vi "Setting_Command_List.vi"(8 "error in (no error)":errorcluster, 11 "VISA resource name":refnum<visa-resource-name>) -> (0 "error out":errorcluster, 2 "read buffer":string, 3 "VISA resource name out":refnum<visa-resource-name>)   [LabVIEW 2020]
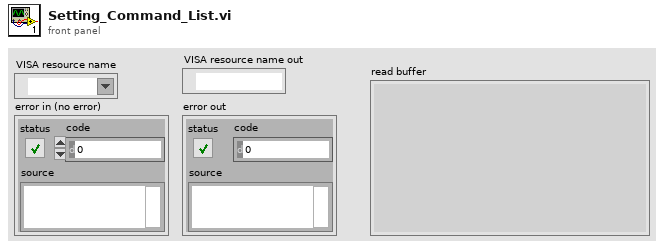
[diagram p1: front panel]
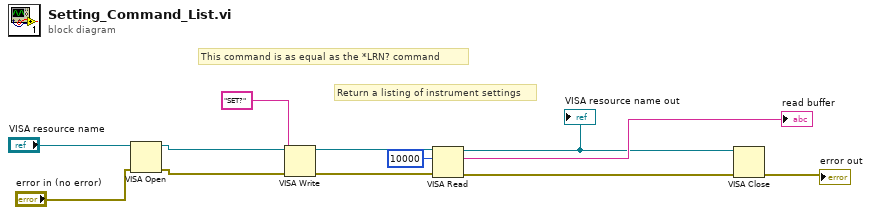
[diagram p0: block diagram]
diagram:
  # "This command is as equal as the *LRN? command"
  # "Return a listing of instrument settings"
  n1 = VISA Open(error in (no error)="error in (no error)", VISA resource name="VISA resource name") -> (VISA resource name=w3:refnum<visa-resource-name>, error out=w1:errorcluster)  [unwired: 3 in]
  n2 = VISA Write(VISA resource name=w3, write buffer="SET?", error in (no error)=w1) -> (VISA resource name out=w11:refnum<visa-resource-name>, error out=w10:errorcluster)  [unwired: 1 out]
  n3 = VISA Read(VISA resource name=w11, byte count=u32 10000, error in (no error)=w10) -> (VISA resource name out=w7:refnum<visa-resource-name>, read buffer=→"read buffer":string, error out=w6:errorcluster)  [unwired: 1 out]
  "VISA resource name out" <- w7
  n4 = VISA Close(VISA resource name=w7, error in (no error)=w6) -> (error out=→"error out":errorcluster)
